vi "Mark Favorite.vi"(8 "error in (no error)":errorcluster, 10 "Favorite?":bool, 11 "ID":u32) -> (0 "error out":errorcluster, 3 "dup ID":u32)   [LabVIEW 2014, in "Contact Data.lvlib"]
doc: "Marks or unmarks a single contact as being a favorite in the address book data store."
uses:
  Contact Data.lvlib
  Position.ctl
  Contact.ctl
  Command.ctl
  Controls.ctl
  DesinationControls.ctl
  DestinationCluster.ctl
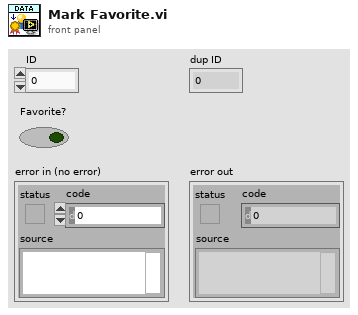
[diagram p1: front panel]
types:
  T1 = typedef "Contact Data.lvlib/Command.ctl" = enum16{"Load", "Save", "Get All Data", "Get Single Data", "Set Single Data", "Set Single Data (Check)", "Remove Single Data", "Set Favorite Status", "Is Data Modified", "Import Data"}
  T2 = typedef "Contact Data.lvlib/Contact.ctl" = cluster{"ID":u32, "UUID":string, "Name":string, "Iteration":i32, "Posit Array":T3[], "Controls":T4, "DestArray":T5[], "SetSpeed":dbl, "Speed":dbl}
  T3 = typedef "Contact Data.lvlib/Position.ctl" = cluster{"X":dbl, "Y":dbl, "Z":dbl}
  T4 = typedef "Contact Data.lvlib/Controls.ctl" = cluster{"throttle":dbl, "brake":dbl, "horn":dbl, "wait":dbl}
  T5 = typedef "Contact Data.lvlib/DestinationCluster.ctl" = cluster{"Desination":string, "DestControls":T6, "Timer":u32, "Set Timer":u32, "Time Stamp":timestamp, "Repeat?":bool, "Optional Data":string, "Distance":dbl}
  T6 = typedef "Contact Data.lvlib/DesinationControls.ctl" = enum16{"Tracker", "Manual", "Stop", "Station DateTime", "Station Timer", "Maintain"}
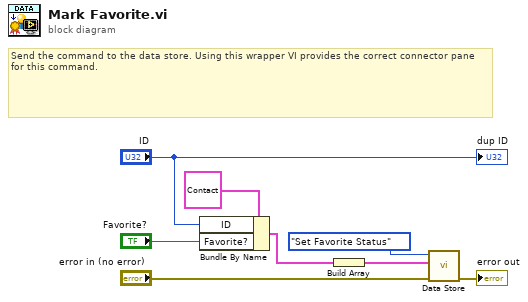
[diagram p0: block diagram]
diagram:
  # "Send the command to the data store. Using this wrapper VI provides the correct connector pane for this command."
  n1 = Bundle By Name(cluster=T2 {"ID"=0, "UUID"="", "Name"="", "Iteration"=0, "Posit Array"=[], "Controls"={"throttle"=0.0, "brake"=0.0, "horn"=0.0, "wait"=0.5}, "DestArray"=[], "SetSpeed"=0.0, "Speed"=0.0} ("Contact"), "ID"="ID", "Favorite?"="Favorite?") -> (w6:T2)
  n2 = Build Array(w6) -> (w1:T2[])
  n3 = call "Data Store.vi"("error in (no error)"="error in (no error)", "Contact in"=w1, "Command"=Command."Set Favorite Status") -> ("error out"=→"error out":errorcluster)  [unwired: 6 in, 2 out]
  "dup ID" <- "ID"
